vi "Untitled 1 (SubVI).vi"(11 "Response body":string) -> (1 "Cluster 3":cluster{dbl[], dbl[]}, 2 "Cluster":cluster{dbl, dbl}, 3 "Cluster 2":cluster{dbl, dbl}, 4 "Gauge":dbl(knob) scale=0.0..360.0, 5 "angle":dbl, 6 "Przeszkoda":dbl)   [LabVIEW 2024]
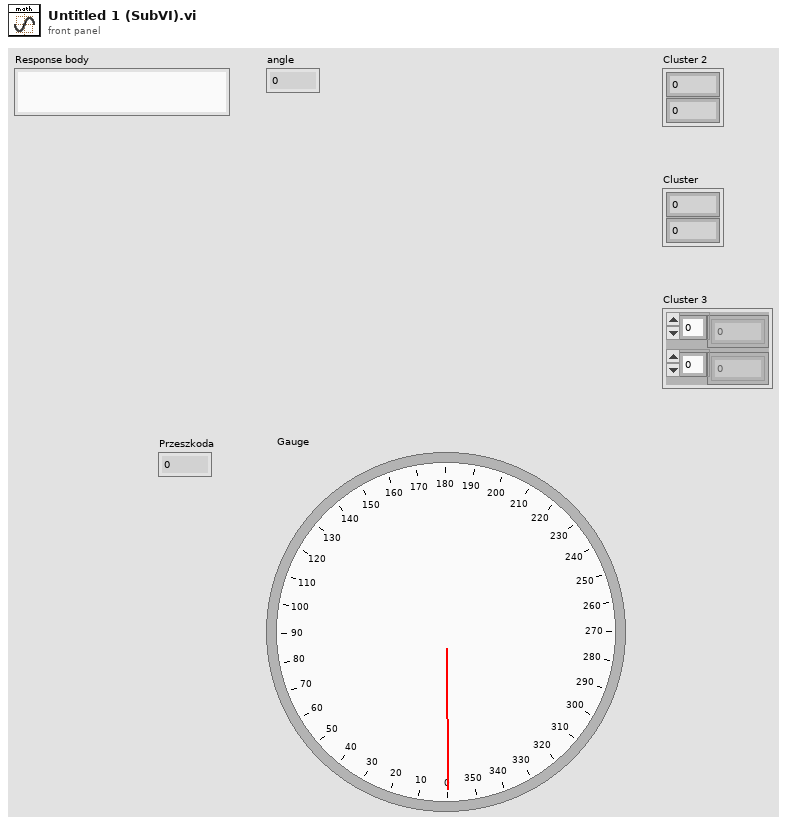
[diagram p1: front panel]
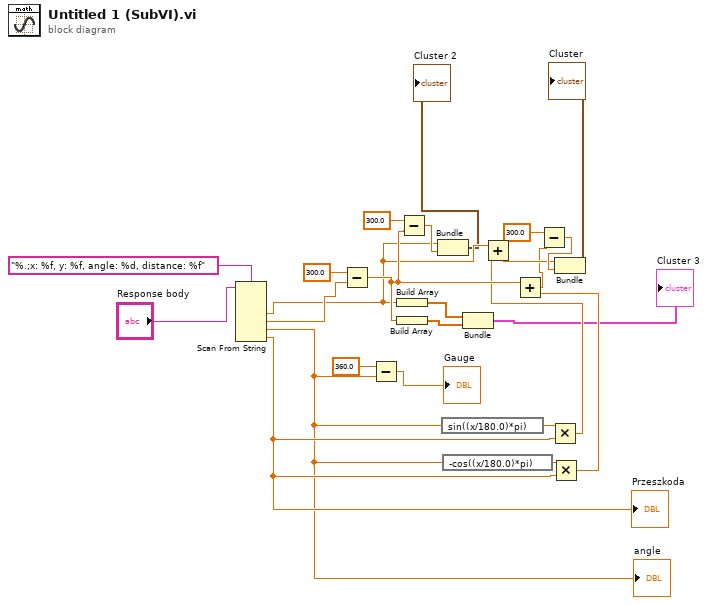
[diagram p0: block diagram]
diagram:
  n1 = Scan From String(format string="%.;x: %f, y: %f, angle: %d, distance: %f", input string="Response body") -> (output 1=w13:dbl, output 2=w19:dbl, output 3=w2:dbl, output 4=w20:dbl)  [unwired: 6 in, 3 out]
  "angle" <- w2
  "Przeszkoda" <- w20
  n2 = Subtract(x=300.0, y=w19) -> (x-y=w22:dbl)
  n3 = Subtract(x=360.0, y=w2) -> (x-y=→"Gauge":dbl)
  n4 = Build Array(w13) -> (w6:dbl[])
  n5 = Build Array(w22) -> (w7:dbl[])
  n6 = Subtract(x=300.0, y=w22) -> (x-y=w21:dbl)
  n7 = Bundle(w13, w21) -> (→"Cluster 2":cluster{dbl, dbl})  [unwired: 1 in]
  n8 = expression code="sin((x/180.0)*pi)" ("degrees to radians")(w2) -> (w14:dbl)
  n9 = expression code="-cos((x/180.0)*pi)" ("degrees to radians")(w2) -> (w15:dbl)
  n10 = Bundle(w6, w7) -> (→"Cluster 3":cluster{dbl[], dbl[]})  [unwired: 1 in]
  n11 = Multiply(x=w14, y=w20) -> (x*y=w16:dbl)
  n12 = Add(x=w13, y=w16) -> (x+y=w12:dbl)
  n13 = Multiply(x=w15, y=w20) -> (x*y=w17:dbl)
  n14 = Add(x=w22, y=w17) -> (x+y=w4:dbl)
  n15 = Subtract(x=300.0, y=w4) -> (x-y=w25:dbl)
  n16 = Bundle(w12, w25) -> (→"Cluster":cluster{dbl, dbl})  [unwired: 1 in]
